vi "Send LogStatementMsg.vi"(8 "error in (no error)":errorcluster, 10 "Statement":T1={"timestamp"=timestamp(0 s since 1904-01-01), "level"=enum."INFO", "sourceTag"="", "originVI"="", "message"=""}, 11 "Enqueuer in":refnum<class "Message Enqueuer.lvclass">) -> (0 "error out":errorcluster, 3 "Enqueuer out":refnum<class "Message Enqueuer.lvclass">)   [LabVIEW 2026, in "Lumberjack.lvlib" / "LogStatementMsg.lvclass"]
doc: "Constructs a LogStatementMsg wrapping one Statement and enqueues it to a target actor.\nThe hot-path carrier: the appender's Do gates the Statement (threshold then filter) and writes it to its sink. Community so the log VIs enqueue it directly.\nLumberjack.lvlib, LogStatementMsg.lvclass, community (friend within the library)."
uses:
  LogStatementMsg.lvclass
  TypeDefs/Statement.ctl
  TypeDefs/Severity.ctl
  <vilib>/ActorFramework/Message Enqueuer/Message Enqueuer.lvclass
  <vilib>/ActorFramework/Message Enqueuer/Message Enqueuer.lvclass/Message Enqueuer.ctl
  <vilib>/ActorFramework/Message Priority Queue/Priority Enqueue.vi
  Lumberjack.lvlib
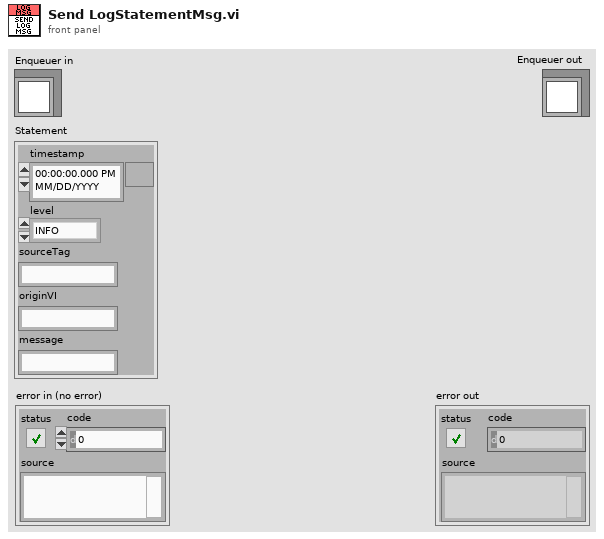
[diagram p1: front panel]
types:
  T1 = typedef "Lumberjack.lvlib/Statement.ctl" = cluster{"timestamp":timestamp, "level":T2, "sourceTag":string, "originVI":string, "message":string}
  T2 = typedef "Lumberjack.lvlib/Severity.ctl" = enum16{"OFF", "FATAL", "ERROR", "WARN", "INFO", "DEBUG", "TRACE", "ALL"}
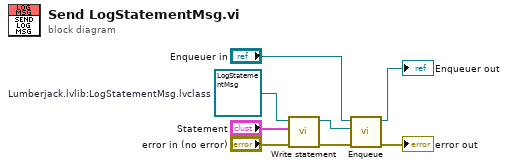
[diagram p0: block diagram]
diagram:
  w1 = refnum<class "LogStatementMsg.lvclass"> refnum  # Lumberjack.lvlib:LogStatementMsg.lvclass
  n1 = call-dynamic "Write statement.vi"("error in (no error)"="error in (no error)", "Statement"="Statement", "LogStatementMsg in"=w1) -> ("error out"=w4:errorcluster, "LogStatementMsg out"=w3:refnum<class "LogStatementMsg.lvclass">)  [unwired: 7 in]
  n2 = call <vilib>:"Enqueue.vi"("error in (no error)"=w4, "Message"=w3, "Message Enqueuer in"="Enqueuer in") -> ("error out"=→"error out":errorcluster, "Message Enqueuer out"=→"Enqueuer out":refnum<class "Message Enqueuer.lvclass">)  [unwired: 7 in]
